vi "Write Update Fan Status Message.vi"(10 "Update Msg":refnum<class "Update Fan Status Msg.lvclass">, 11 "Dual Fan in":refnum<class "Dual Fan.lvclass">) -> (3 "Dual Fan out":refnum<class "Dual Fan.lvclass">)   [LabVIEW 2025, in "Dual Fan.lvlib" / "Dual Fan.lvclass"]
doc: "Writes the message object to use for sending fan status updates to the caller. Callers should set this value *before* calling Launch Actor.vi."
uses:
  Dual Fan.lvclass
  Update Fan Status Msg/Update Fan Status Msg.lvclass
  Dual Fan.lvclass/Dual Fan.ctl
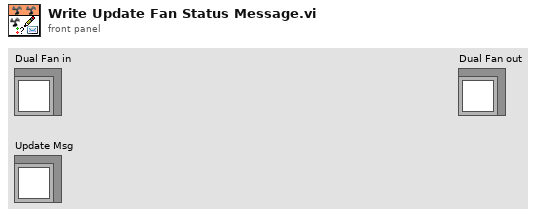
[diagram p1: front panel]
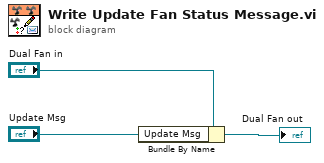
[diagram p0: block diagram]
diagram:
  n1 = Bundle By Name(cluster="Dual Fan in", "Update Msg"="Update Msg") -> (→"Dual Fan out":refnum<class "Dual Fan.lvclass">)
